vi "PCO_SetStorageStruct.vi"(8 "error in (no error)":errorcluster {"code" format="%x"}, 10 "strStorage":T1, 11 "ph":u64) -> (0 "error out":errorcluster {"code" format="%x"}, 2 "ErrorMessage":i32 format="%x", 3 "ph out":u64)   [LabVIEW 2019, in "SDK.lvlib" / "StorageControl.lvlib"]
doc: "<b>Description:</b>\nThis function does set the complete set of storage settings at once. For the sake of clarity it is better to use the functions which change distinct parameter despite changing all settings at once.\nAn invalid value for one of the parameter will result in a failure response message.\nThe command will be rejected, if Recording State is [run], see PCO_GetRecordingState.\n\n<b>Supported camera type:</b>\npco.dimax, pco.1200, pco.1600, pco.2000, pco.4000\n\n<b>Descriptor dependency:</b>\ndwGeneralCapsDESC1: NO_RECORDER"
uses:
  StorageControl.lvlib
  Structures/Structures.lvlib
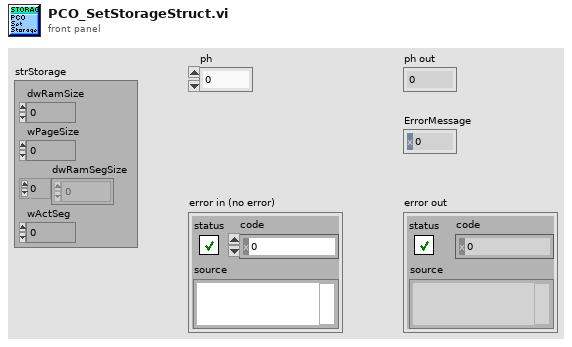
[diagram p1: front panel]
types:
  T1 = cluster{"dwRamSize":u32, "wPageSize":u16, "dwRamSegSize":u32[], "wActSeg":u16}
  T2 = cluster{"wSize":u16, "ZZwAlignDummy1":u16, "dwRamSize":u32, "wPageSize":u16, "ZZwAlignDummy4":u16, "dwRamSegSize":cluster{u32, u32, u32, u32}, "ZZdwDummyrs":cluster{u32, u32, u32, u32, u32, u32, u32, u32, u32, u32, u32, u32, u32, u32, u32, u32, u32, u32, u32, u32}, "wActSeg":u16, "ZZwDummy":cluster{u16, u16, u16, u16, u16, u16, u16, u16, u16, u16, u16, u16, u16, u16, u16, u16, u16, u16, u16, u16, u16, u16, u16, u16, u16, u16, u16, u16, u16, u16, u16, u16, u16, u16, u16, u16, u16, u16, u16}}
  T3 = cluster{u32, u32, u32, u32, u32, u32, u32, u32, u32, u32, u32, u32, u32, u32, u32, u32, u32, u32, u32, u32}
  T4 = cluster{u16, u16, u16, u16, u16, u16, u16, u16, u16, u16, u16, u16, u16, u16, u16, u16, u16, u16, u16, u16, u16, u16, u16, u16, u16, u16, u16, u16, u16, u16, u16, u16, u16, u16, u16, u16, u16, u16, u16}
  T5 = cluster{"dwRamSegSize[0]":u32, "dwRamSegSize[1]":u32, "dwRamSegSize[2]":u32, "dwRamSegSize[3]":u32}
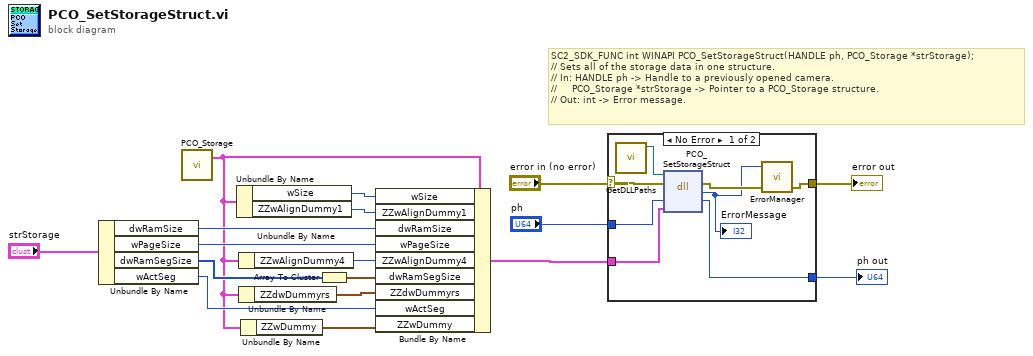
[diagram p0: block diagram]
diagram:
  # "SC2_SDK_FUNC int WINAPI PCO_SetStorageStruct(HANDLE ph, PCO_Storage *strStorage);\n// Sets all of the storage data in one structure.\n// In: HANDLE ph -> Handle to a previously opened camera.\n//     PCO_Storage *strStorage -> Pointer to a PCO_Storage structure.\n// Out: int -> Error message."
  n1 = Unbundle By Name("strStorage") -> ("dwRamSize"=w10:u32, "wPageSize"=w9:u16, "dwRamSegSize"=w7:u32[], "wActSeg"=w5:u16)
  n2 = call "PCO_Storage.vi"() -> ("PCO_Storage_Raw"=w3:T2)  [unwired: 4 in, 3 out]
  n3 = Unbundle By Name(w3) -> ("wSize"=w12:u16, "ZZwAlignDummy1"=w11:u16)
  n4 = Unbundle By Name(w3) -> ("ZZwAlignDummy4"=w8:u16)
  n5 = Unbundle By Name(w3) -> ("ZZdwDummyrs"=w4:T3)
  n6 = Unbundle By Name(w3) -> ("ZZwDummy"=w2:T4)
  n7 = Array To Cluster(array=w7) -> (cluster=w6:T5)
  n8 = Bundle By Name(cluster=w3, "wSize"=w12, "ZZwAlignDummy1"=w11, "dwRamSize"=w10, "wPageSize"=w9, "ZZwAlignDummy4"=w8, "dwRamSegSize"=w6, "ZZdwDummyrs"=w4, "wActSeg"=w5, "ZZwDummy"=w2) -> (w1:T2)
  n9 = case shown="No Error" "error in (no error)" {
    selector: "error in (no error)" -> [w22 w27]
    tunnel: "ph" -> [w25 w26]
    tunnel: [w24 w26] -> w16
    tunnel: w1 -> [w23 _]
    tunnel: [w20 w27] -> w15
    frame No Error {
      n10 = call "GetDLLPaths.vi"() -> ("SC2_Cam_Path"=w18:path)  [unwired: 8 in, 3 out]
      n11 = dll-call lib="?" fn="PCO_SetStorageStruct"(path in=w18, error in=w22, "ph"=w25, "strStorage"=w23) -> (error out=w21:errorcluster, "return type"=w19:i32, "ph"=w24:u64)  [unwired: 2 in, 1 out]
      "ErrorMessage" <- w19
      n12 = call "ErrorManager.vi"("error in (no error)"=w21, "error code"=w19) -> ("error out"=w20:errorcluster)  [unwired: 2 in, 1 out]
    }
    frame Error {
    }
  }
  "ph out" <- w16
  "error out" <- w15
